vi "S2C_VLFT10_Proc_GetSoftwareState.vi"(7 "Timeout":dbl, 8 "Error In":errorcluster, 11 "State":string) -> (0 "Error Out":errorcluster, 3 "Result":string)   [LabVIEW 2015]
uses:
  Fornax/VIs/PolyDriver/Typedefs/SwUpdateState.ctl
  Fornax/VIs/PolyDriver/Typedefs/SystemState.ctl
  Fornax/VIs/S2C_FORNAX_Proc_Globals.vi
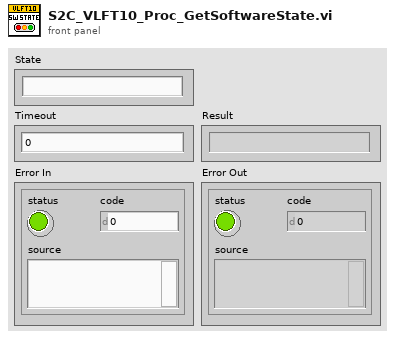
[diagram p1: front panel]
types:
  T1 = typedef "SwUpdateState.ctl" = i16
  T2 = cluster{"SwUpdateState":T1, "PostDelay (ms)":i32, "ClearFornaxMsgs":bool}
  T3 = cluster{"Partition":string, "Message":string, "M_SwUpdateState":T1, "M_ProgressStep":i32, "M_ProgressMaximum":i32, "M_ProgressMessage":string, "M_OperationProgressStep":i32, "M_OperationProgressMaximum":i32, "M_OperationProgressMessage":string, "M_Crc32":i32}
  T4 = cluster{"Partition":string, "Message":string, "M_SwUpdateState":T1, "M_ProgressStep":i32, "M_ProgressMaximum":i32, "M_ProgressMessage":string, "M_OperationProgressStep":i32, "M_OperationProgressMaximum":i32, "M_OperationProgressMessage":string}
  T5 = typedef "SystemState.ctl" = i16
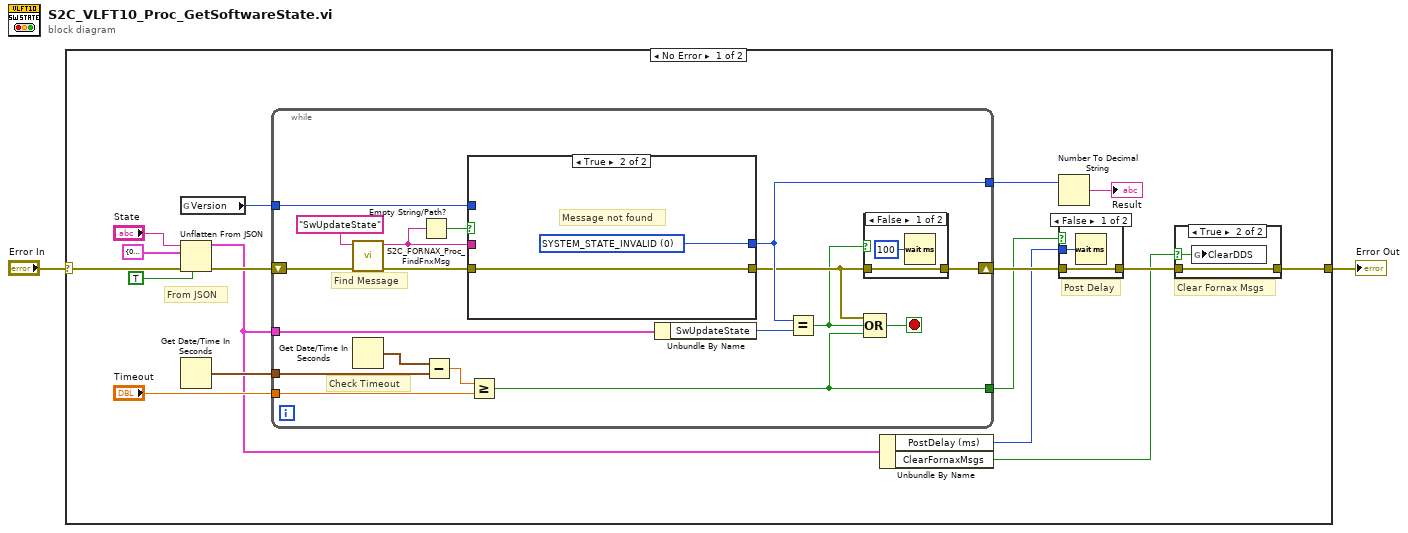
[diagram p0: block diagram]
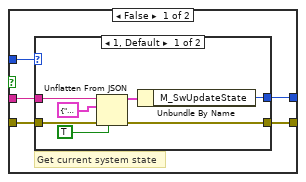
[diagram p5: hidden frame]
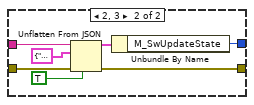
[diagram p6: hidden frame]
diagram:
  n1 = case shown="No Error" "Error In" {
    selector: "Error In" -> [w16 w68]
    tunnel: [w5 w68] -> w1
    frame No Error {
      # "Clear Fornax Msgs"
      # "Post Delay"
      # "From JSON"
      n2 = global read "S2C_FORNAX_Proc_Globals.vi" "Version"() -> (w19:i32)
      n3 = Unflatten From JSON(JSON string="State", type and defaults=T2 {"SwUpdateState"=0, "PostDelay (ms)"=0, "ClearFornaxMsgs"=FALSE}, default null elements? (F)=TRUE, error in (no error)=w16) -> (value=w10:T2, error out=w15:errorcluster)  [unwired: 3 in]
      n4 = Get Date/Time In Seconds() -> (seconds since 1Jan1904=w14:timestamp)
      n5 = while {
        tunnel: w19 -> [w41]
        tunnel: w10 -> [w39]
        shift-right: [w28] -> w9
        shift-left: w15 -> [w40]
        tunnel: w14 -> [w35]
        tunnel: "Timeout" -> [w34]
        tunnel: [w30] -> w12
        tunnel: [w26] -> w8
        stop <- w31 stop-if-true
        # "Check Timeout"
        # "Find Message"
        n6 = call "S2C_FORNAX_Proc_FindFnxMsg.vi"("Error In"=w40, "MsgName"="SwUpdateState") -> ("Error Out"=w43:errorcluster, "Message"=w37:string)  [unwired: 8 in]
        n7 = Get Date/Time In Seconds() -> (seconds since 1Jan1904=w36:timestamp)
        n8 = Empty String/Path?(string/path=w37) -> (empty?=w38:bool)
        n9 = Subtract(x=w36, y=w35) -> (x-y=w33:dbl)
        n10 = case shown="True" w38 {
          tunnel: w43 -> [w51 w67]
          tunnel: w41 -> [w50 _]
          tunnel: [w49 w67] -> w29
          tunnel: [w48 w66] -> w30
          tunnel: w37 -> [w47 _]
          frame False {
            # "Get current system state"
            n11 = case shown="1, Default" w50 {
              tunnel: w51 -> [w57 w64]
              tunnel: [w55 w62] -> w49
              tunnel: [w54 w61] -> w48
              tunnel: w47 -> [w53 w60]
              frame 1, Default {
                n12 = Unflatten From JSON(JSON string=w53, type and defaults=T3 {"Partition"="", "Message"="", "M_SwUpdateState"=0, "M_ProgressStep"=0, "M_ProgressMaximum"=0, "M_ProgressMessage"="", "M_OperationProgressStep"=0, "M_OperationProgressMaximum"=0, "M_OperationProgressMessage"="", "M_Crc32"=0}, default null elements? (F)=TRUE, error in (no error)=w57) -> (value=w56:T3, error out=w55:errorcluster)  [unwired: 3 in]
                n13 = Unbundle By Name(w56) -> ("M_SwUpdateState"=w54:T1)
              }
              frame 2, 3 {
                n14 = Unflatten From JSON(JSON string=w60, type and defaults=T4 {"Partition"="", "Message"="", "M_SwUpdateState"=0, "M_ProgressStep"=0, "M_ProgressMaximum"=0, "M_ProgressMessage"="", "M_OperationProgressStep"=0, "M_OperationProgressMaximum"=0, "M_OperationProgressMessage"=""}, default null elements? (F)=TRUE, error in (no error)=w64) -> (value=w63:T4, error out=w62:errorcluster)  [unwired: 3 in]
                n15 = Unbundle By Name(w63) -> ("M_SwUpdateState"=w61:T1)
              }
            }
          }
          frame True {
            w66 = T5 0 items=["SYSTEM_STATE_INVALID", "SYSTEM_STATE_INIT", "SYSTEM_STATE_POST", "SYSTEM_STATE_CLINICAL", "SYSTEM_STATE_SERVICE", "SYSTEM_STATE_SW_UPDATE", "SYSTEM_STATE_SHUTDOWN", "SYSTEM_STATE_CALIBRATION", "SYSTEM_STATE_CONFIGURATION", "SYSTEM_STATE_CLINICAL_CONFIGURATION"] ("M_SystemState")
            # "Message not found"
          }
        }
        n16 = Greater Or Equal?(x=w33, y=w34) -> (x >= y?=w26:bool)
        n17 = Unbundle By Name(w39) -> ("SwUpdateState"=w32:T1)
        n18 = Equal?(x=w30, y=w32) -> (x = y?=w27:bool)
        n19 = case shown="False" w27 {
          tunnel: w29 -> [w45 w46]
          tunnel: [w45 w46] -> w28
          frame False {
            n20 = Wait (ms)(milliseconds to wait=u32 100) -> ()  [unwired: 1 out]
          }
          frame True {
          }
        }
        n21 = Compound Arithmetic op=OR(w29, w27, w26) -> (w31:bool)
      }
      n22 = Unbundle By Name(w10) -> ("PostDelay (ms)"=w7:i32, "ClearFornaxMsgs"=w4:bool)
      n23 = Number To Decimal String(number=w12) -> (decimal integer string=→"Result":string)  [unwired: 1 in]
      n24 = case shown="False" w8 {
        tunnel: w9 -> [w24 w25]
        tunnel: [w24 w25] -> w6
        tunnel: w7 -> [w23 _]
        frame False {
          n25 = Wait (ms)(milliseconds to wait=w23) -> ()  [unwired: 1 out]
        }
        frame True {
        }
      }
      n26 = case shown="True" w4 {
        selector: w4 -> [_ w21]
        tunnel: w6 -> [w20 w22]
        tunnel: [w20 w22] -> w5
        frame False {
        }
        frame True {
          n27 = global write "S2C_FORNAX_Proc_Globals.vi" "ClearDDS"(w21) -> ()
        }
      }
    }
    frame Error {
    }
  }
  "Error Out" <- w1
